vi "Is Sequence Local.vi"(11 "Terminal in":refnum<vi>) -> (3 "Is Seq Local?":bool)   [LabVIEW 2023]
panel:
  out "error out":errorcluster
  in  "error in":errorcluster
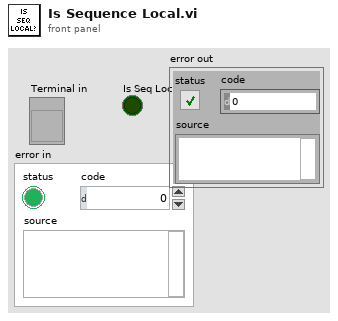
[diagram p1: front panel]
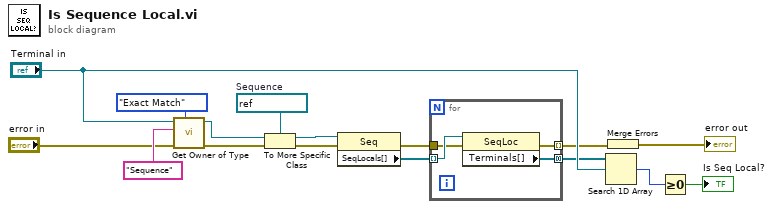
[diagram p0: block diagram]
diagram:
  w9 = refnum<vi> refnum  # Sequence
  n1 = call "Get Owner of Type.vi"("Match Type"=enum16{"Exact Match", "Contains"}."Exact Match", "error in"="error in", "Owner Class Name desired"="Sequence", "reference"="Terminal in") -> ("error out"=w5:errorcluster, "Owner of Type"=w10:refnum<vi>)  [unwired: 3 in, 3 out]
  n2 = To More Specific Class(target class=w9, reference=w10, error in=w5) -> (specific class reference=w11:refnum<vi>, error out=w4:errorcluster)
  n3 = property class="Seq"(reference=w11, error in=w4) -> (error out=w3:errorcluster, "SeqLocals[]"=w15:refnum<vi>[])  [unwired: 1 out]
  n4 = for {
    tunnel: w15 -> [w20] mode=indexing
    tunnel: [w19] -> w12 mode=concatenating
    tunnel: w3 -> [w18]
    tunnel: [w17] -> w2 mode=indexing
    n5 = property class="SeqLoc"(reference=w20, error in=w18) -> (error out=w17:errorcluster, "Terminals[]"=w19:refnum<vi>[])  [unwired: 1 out]
  }
  n6 = Search 1D Array(1D array=w12, element="Terminal in") -> (index of element=w13:i32)  [unwired: 1 in]
  n7 = Merge Errors(w2) -> (→"error out":errorcluster)
  n8 = Greater Or Equal To 0?(x=w13) -> (x >= 0?=→"Is Seq Local?":bool)
